vi "Swerve drive to 4 roues.vi"(11 "SwerveDrive":T2) -> (3 "4 roues":T1 {"ARD"."Vitesse" scale=-1.0..1.0; "ARD"."Angle" scale=-180.0..180.0; "ARG"."Vitesse" scale=-1.0..1.0; "ARG"."Angle" scale=-180.0..180.0; "AVD"."Vitesse" scale=-1.0..1.0; "AVD"."Angle" scale=-180.0..180.0; "AVG"."Vitesse" scale=-1.0..1.0; "AVG"."Angle" scale=-180.0..180.0})   [LabVIEW 2018]
uses:
  Direction 4 roues.ctl
  SwerveDrive.ctl
panel:
  in  "TD":T1 {"ARD"."Vitesse" scale=-1.0..1.0; "ARD"."Angle" scale=-180.0..180.0; "ARG"."Vitesse" scale=-1.0..1.0; "ARG"."Angle" scale=-180.0..180.0; "AVD"."Vitesse" scale=-1.0..1.0; "AVD"."Angle" scale=-180.0..180.0; "AVG"."Vitesse" scale=-1.0..1.0; "AVG"."Angle" scale=-180.0..180.0}
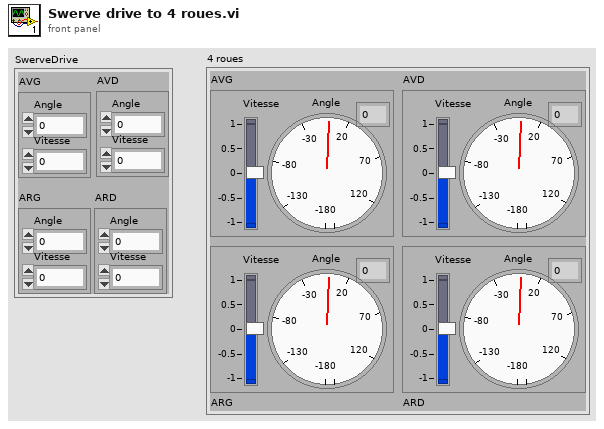
[diagram p1: front panel]
types:
  T1 = typedef "Direction 4 roues.ctl" = cluster{"AVG":cluster{"Angle":dbl, "Vitesse":dbl}, "AVD":cluster{"Angle":dbl, "Vitesse":dbl}, "ARG":cluster{"Angle":dbl, "Vitesse":dbl}, "ARD":cluster{"Angle":dbl, "Vitesse":dbl}}
  T2 = typedef "SwerveDrive.ctl" = cluster{"AVD":cluster{"Angle":dbl, "Vitesse":dbl}, "AVG":cluster{"Angle":dbl, "Vitesse":dbl}, "ARG":cluster{"Angle":dbl, "Vitesse":dbl}, "ARD":cluster{"Angle":dbl, "Vitesse":dbl}}
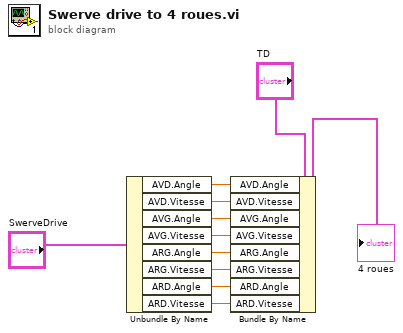
[diagram p0: block diagram]
diagram:
  n1 = Unbundle By Name("SwerveDrive") -> ("AVD.Angle"=w11:dbl, "AVD.Vitesse"=w10:dbl, "AVG.Angle"=w9:dbl, "AVG.Vitesse"=w8:dbl, "ARG.Angle"=w7:dbl, "ARG.Vitesse"=w6:dbl, "ARD.Angle"=w5:dbl, "ARD.Vitesse"=w4:dbl)
  n2 = Bundle By Name(cluster="TD", "AVD.Angle"=w11, "AVD.Vitesse"=w10, "AVG.Angle"=w9, "AVG.Vitesse"=w8, "ARG.Angle"=w7, "ARG.Vitesse"=w6, "ARD.Angle"=w5, "ARD.Vitesse"=w4) -> (→"4 roues":T1)
